vi "FitBothWays.vi"(5 "Fit Zmin":dbl, 7 "Fit Zmax":dbl, 8 "Zref":dbl, 9 "zUCluster in":cluster{"Array":dbl[], "Array":dbl[]}) -> (2 "PowerLawWithDisplacement":T1, 3 "PowerLawNoDisplacement":T1)   [LabVIEW 2021]
uses:
  PowerLaw.ctl
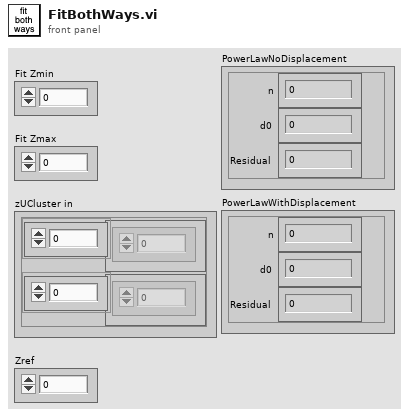
[diagram p1: front panel]
types:
  T1 = typedef "PowerLaw.ctl" = cluster{"n":dbl, "d0":dbl, "Residual":dbl}
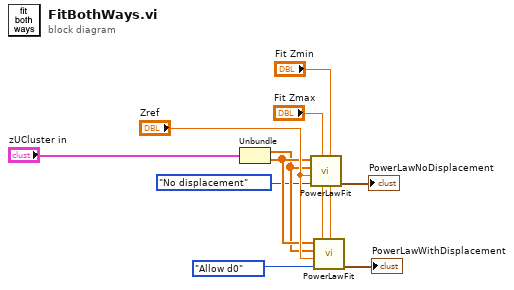
[diagram p0: block diagram]
diagram:
  n1 = Unbundle("zUCluster in") -> ("Array"=w2:dbl[], "Array"=w3:dbl[])
  n2 = call "PowerLawFit.vi"("MinFitZ"="Fit Zmin", "MaxFitZ"="Fit Zmax", "ZeroDisplacement?"=enum16{"Allow d0", "No displacement"}."No displacement", "Zref"="Zref", "U/Uref"=w2, "z"=w3) -> ("PowerLaw"=→"PowerLawNoDisplacement":T1)  [unwired: 2 in, 3 out]
  n3 = call "PowerLawFit.vi"("MinFitZ"="Fit Zmin", "MaxFitZ"="Fit Zmax", "ZeroDisplacement?"=enum16{"Allow d0", "No displacement"}."Allow d0", "Zref"="Zref", "U/Uref"=w2, "z"=w3) -> ("PowerLaw"=→"PowerLawWithDisplacement":T1)  [unwired: 2 in, 3 out]
